vi "createQuery.vi"(8 "error in (no error)":errorcluster, 9 "id":T1, 10 "CoolerQuery":T2=enum."ReadControlSensor", 11 "CoolerSerialCommand in":refnum<class "CoolerSerialCommand.lvclass">) -> (0 "error out":errorcluster, 2 "SerialQueryStr":string, 3 "CoolerSerialCommand out":refnum<class "CoolerSerialCommand.lvclass">)   [LabVIEW 2016, in "CoolerSerialCommand.lvclass"]
uses:
  CoolerSerialCommand.lvclass
  typedefs/CoolerQuery.ctl
  typedefs/CoolerId.ctl
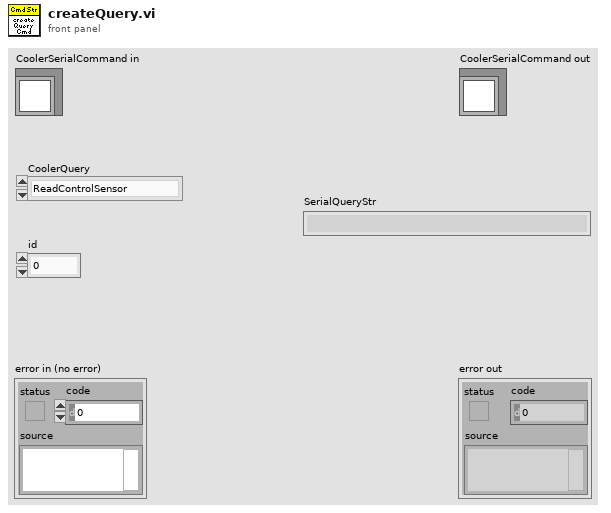
[diagram p1: front panel]
types:
  T1 = typedef "CoolerId.ctl" = u16
  T2 = typedef "CoolerQuery.ctl" = enum16{"ReadSerialWatchdog", "ReadControlSensor", "ReadSetTemperature", "ReadSupplyTemperature", "ReadExternalRTD", "ReadExternalThermistor", "ReadReturnTemperature", "ReadAmbientTemperature", "ReadProcessFlow", "ReadTECBank1Current", "ReadTECBank2Current", "ReadTEDriveLevel", "ReadAlarmStateLevel1", "ReadAlarmStateLevel21", "ReadAlarmStateLevel22", "ReadWarningStateLevel1", "ReadHighSupplyTempWarning", "ReadLowSupplyTempWarning", "ReadHighAmbientTempWarning", "ReadLowAmbientTempWarning", "ReadLowProcessFlowWarning", "ReadHighSupplyTempAlarm", "ReadLowSupplyTempAlarm", "ReadHighAmbientTempAlarm", "ReadLowAmbientTempAlarm", "ReadLowProcessFlowAlarm", "ReadPWMandRelayStatus", "ReadPIDStatus", "ReadUnitUpTime", "ReadFan1Speed", "ReadFan2Speed", "ReadFan3Speed", "ReadFan4Speed"}
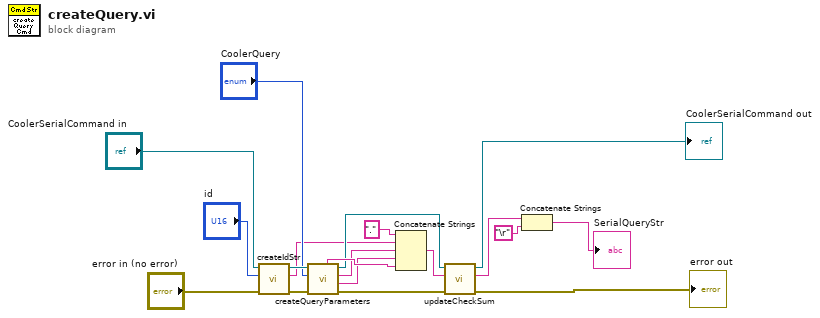
[diagram p0: block diagram]
diagram:
  n1 = call "createIdStr.vi"("error in (no error)"="error in (no error)", "id"="id", "CoolerSerialCommand in"="CoolerSerialCommand in") -> ("error out"=w11:errorcluster, "idStr"=w2:string, "CoolerSerialCommand out"=w13:refnum<class "CoolerSerialCommand.lvclass">)  [unwired: 6 in]
  n2 = call "createQueryParameters.vi"("error in (no error)"=w11, "CoolerQuery"="CoolerQuery", "CoolerSerialCommand in"=w13) -> ("error out"=w8:errorcluster, "commandName"=w4:string, "commandId"=w5:string, "CoolerSerialCommand out"=w9:refnum<class "CoolerSerialCommand.lvclass">, "cmdData"=w10:string)  [unwired: 4 in]
  n3 = Concatenate Strings("." ("string"), w2, w5, w4, w10) -> (w3:string)
  n4 = call "updateCheckSum.vi"("error in (no error)"=w8, "message"=w3, "CoolerSerialCommand in"=w9) -> ("error out"=→"error out":errorcluster, "result message"=w7:string, "CoolerSerialCommand out"=→"CoolerSerialCommand out":refnum<class "CoolerSerialCommand.lvclass">)  [unwired: 6 in]
  n5 = Concatenate Strings(w7, "\r") -> (→"SerialQueryStr":string)
